vi "waypoints from vision.vi"() -> ()   [LabVIEW 2018]
panel:
  out "Waypoints":dbl[][](array[numeric])
  in  "End Weight":dbl
  in  "Start Weight":dbl
  out "XY Graph":cluster{dbl[], dbl[]}[](graph)
  in  "Vision Data":dbl[](array[numeric]) format="%#_13g"
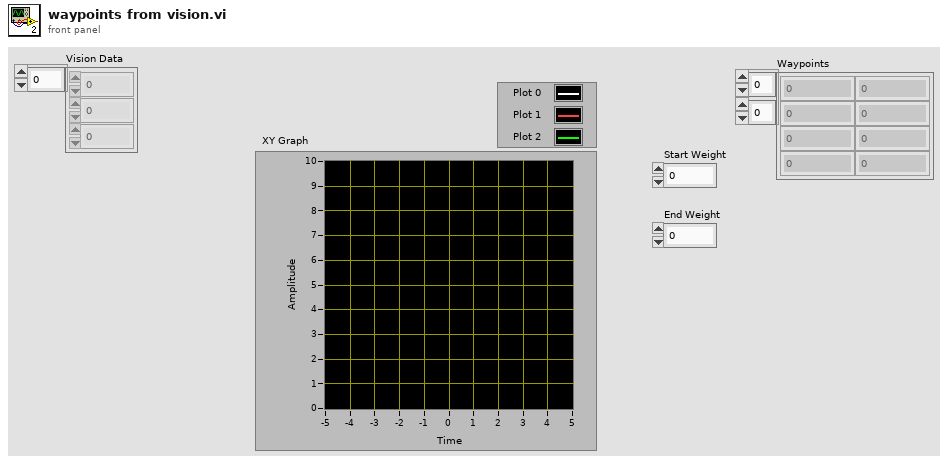
[diagram p1: front panel]
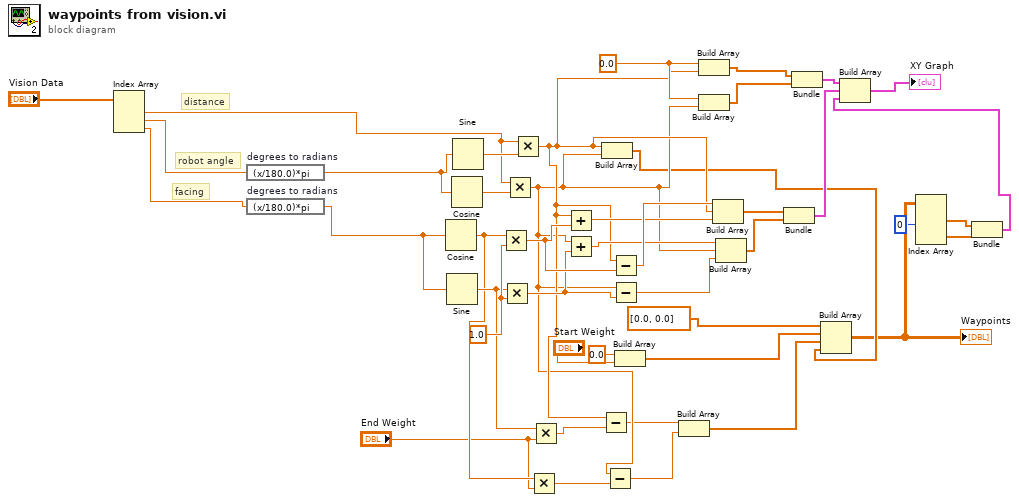
[diagram p0: block diagram]
diagram:
  w31 = 1.0
  w36 = 0.0
  # "facing"
  # "robot angle"
  # "distance"
  n1 = Index Array(array="Vision Data") -> (element #1=w37:dbl, element #2=w42:dbl, element #3=w41:dbl)  [unwired: 3 in]
  n2 = expression code="(x/180.0)*pi" "degrees to radians"(w42) -> (w40:dbl)
  n3 = expression code="(x/180.0)*pi" "degrees to radians"(w41) -> (w32:dbl)
  n4 = Cosine(x=w32) -> (cos(x)=w17:dbl)
  n5 = Sine(x=w32) -> (sin(x)=w18:dbl)
  n6 = Cosine(x=w40) -> (cos(x)=w38:dbl)
  n7 = Sine(x=w40) -> (sin(x)=w39:dbl)
  n8 = Multiply(x=w17, y=w31) -> (x*y=w30:dbl)
  n9 = Multiply(x=w18, y=w31) -> (x*y=w29:dbl)
  n10 = Multiply(x=w37, y=w38) -> (x*y=w12:dbl)
  n11 = Multiply(x=w37, y=w39) -> (x*y=w13:dbl)
  n12 = Multiply(x=w17, y="End Weight") -> (x*y=w14:dbl)
  n13 = Multiply(x=w18, y="End Weight") -> (x*y=w15:dbl)
  n14 = Add(x=w13, y=w30) -> (x+y=w23:dbl)
  n15 = Add(x=w12, y=w29) -> (x+y=w22:dbl)
  n16 = Subtract(x=w13, y=w15) -> (x-y=w11:dbl)
  n17 = Build Array(w13, w12) -> (w6:dbl[])
  n18 = Subtract(x=w12, y=w14) -> (x-y=w10:dbl)
  n19 = Subtract(x=w13, y=w30) -> (x-y=w24:dbl)
  n20 = Subtract(x=w12, y=w29) -> (x-y=w21:dbl)
  n21 = Build Array(0.0 ("element"), "Start Weight") -> (w8:dbl[])
  n22 = Build Array(w11, w10) -> (w7:dbl[])
  n23 = Build Array(w36, w13) -> (w35:dbl[])
  n24 = Build Array(w36, w12) -> (w34:dbl[])
  n25 = Build Array(w24, w13, w23) -> (w28:dbl[])
  n26 = Build Array(w22, w12, w21) -> (w27:dbl[])
  n27 = Bundle(w28, w27) -> (w25:cluster{dbl[], dbl[]})  [unwired: 1 in]
  n28 = Bundle(w35, w34) -> (w33:cluster{dbl[], dbl[]})  [unwired: 1 in]
  n29 = Build Array(dbl[] [0.0, 0.0], w8, w7, w6) -> (w5:dbl[][])
  "Waypoints" <- w5
  n30 = Index Array(array=w5, index (col) #1=0 ("disabled index (col)")) -> (element #1=w4:dbl[], element #2=w3:dbl[])  [unwired: 3 in]
  n31 = Bundle(w4, w3) -> (w2:cluster{dbl[], dbl[]})  [unwired: 1 in]
  n32 = Build Array(w33, w25, w2) -> (→"XY Graph":cluster{dbl[], dbl[]}[])
